vi "rvc Generate polynomial trajectory.vi"(6 "final velocity":dbl, 7 "initial velocity":dbl, 9 "number of timesteps":dbl, 10 "final position":dbl, 11 "initial position":dbl) -> (1 "accelaration":cluster{"time":dbl[], "velocity":dbl[]}(graph), 2 "velocity":cluster{"time":dbl[], "velocity":dbl[]}(graph), 3 "position":cluster{"time":dbl[], "position":dbl[]}(graph))   [LabVIEW 2017]
uses:
  <vilib>/Analysis/1siggen.llb/Ramp Pattern by Samples.vi
  <vilib>/Analysis/polynomials.llb/1D Polynomial Evaluation (DBL).vi
  <vilib>/Analysis/NI_AALBase.lvlib
  <vilib>/Analysis/NI_AALPro.lvlib
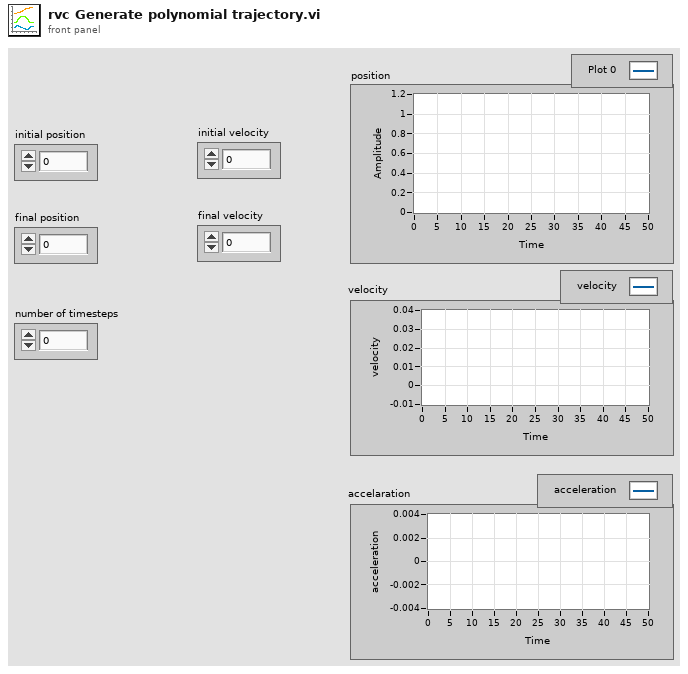
[diagram p1: front panel]
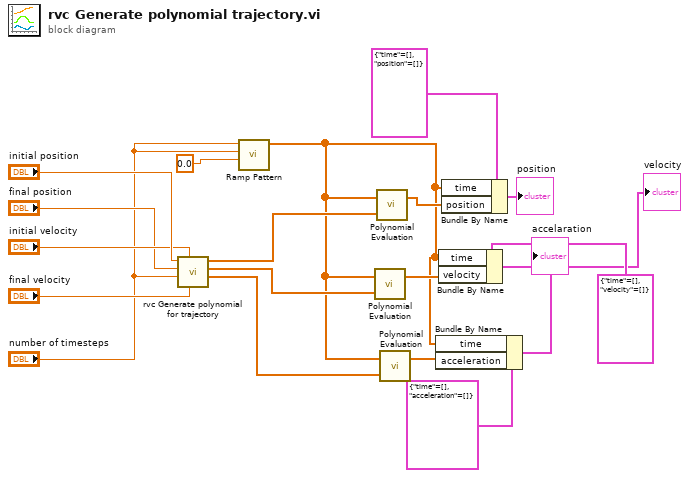
[diagram p0: block diagram]
diagram:
  n1 = call "rvc Generate polynomial for trajectory.vi"("final velocity"="final velocity", "initial velocity"="initial velocity", "number of points"="number of timesteps", "final position"="final position", "initial position"="initial position") -> ("ddcoeff"=w13:dbl[], "dcoeff"=w16:dbl[], "coeff"=w17:dbl[])  [unwired: 4 in]
  n2 = call-poly <vilib>:"Ramp Pattern.vi"("start"=0.0, "end"="number of timesteps", "samples"="number of timesteps") -> ("Ramp Pattern"=w3:dbl[])  [unwired: 7 in, 1 out]
  n3 = call-poly <vilib>:"Polynomial Evaluation.vi"("P(x)"=w16, "A"=w3) -> ("P(A)"=w6:dbl[])  [unwired: 1 out]
  n4 = call-poly <vilib>:"Polynomial Evaluation.vi"("P(x)"=w17, "A"=w3) -> ("P(A)"=w10:dbl[])  [unwired: 1 out]
  n5 = call-poly <vilib>:"Polynomial Evaluation.vi"("P(x)"=w13, "A"=w3) -> ("P(A)"=w7:dbl[])  [unwired: 1 out]
  n6 = Bundle By Name(cluster=cluster{"time":dbl[], "acceleration":dbl[]} {"time"=[], "acceleration"=[]} ("input cluster"), "time"=w3, "acceleration"=w7) -> (→"accelaration":cluster{"time":dbl[], "acceleration":dbl[]})
  n7 = Bundle By Name(cluster=cluster{"time":dbl[], "velocity":dbl[]} {"time"=[], "velocity"=[]} ("input cluster"), "time"=w3, "velocity"=w6) -> (→"velocity":cluster{"time":dbl[], "velocity":dbl[]})
  n8 = Bundle By Name(cluster=cluster{"time":dbl[], "position":dbl[]} {"time"=[], "position"=[]} ("input cluster"), "time"=w3, "position"=w10) -> (→"position":cluster{"time":dbl[], "position":dbl[]})
